vi "sanitize_io.vi"(9 "min":i32, 10 "max":i32=60000, 11 "Input":i32) -> (3 "Sanitized Input":i32)   [LabVIEW 2019]
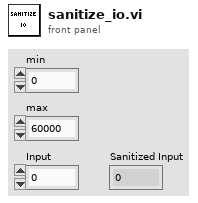
[diagram p1: front panel]
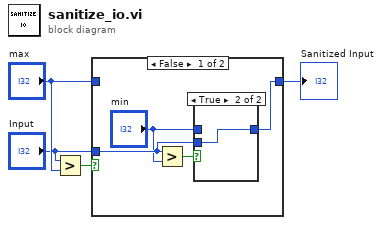
[diagram p0: block diagram]
diagram:
  n1 = Greater?(x="Input", y="max") -> (0:w4:bool)
  n2 = case shown="False" w4 {
    tunnel: [w7 w11] -> w3
    tunnel: "max" -> [_ w11]
    tunnel: "Input" -> [w6 _]
    frame False {
      n3 = Greater?(x=w6, y="min") -> (0:w8:bool)
      n4 = case shown="True" w8 {
        tunnel: [w9 w10] -> w7
        tunnel: w6 -> [_ w10]
        tunnel: "min" -> [w9 _]
        frame False {
        }
        frame True {
        }
      }
    }
    frame True {
    }
  }
  "Sanitized Input" <- w3
